vi "Initialize.vi"(8 "error in":errorcluster, 10 "parameters":variant, 11 "node in":refnum<class "CentralErrorHandler editor node.lvclass">) -> (0 "error out":errorcluster, 2 "summary":T2[](array[typedef]), 3 "data value reference":T1)   [LabVIEW 2017, in "CentralErrorHandler editor node.lvclass"]
doc: "Initializes the data of a node to its default state.\nThe object is not created inside of this VI, because it is created from a File depending on user selection."
uses:
  CentralErrorHandler editor node.lvclass
  C:/Program Files (x86)/National Instruments/LabVIEW 2017/vi.lib/NI/Configuration Framework/Node/NISE_CEF_Node.lvclass
  <vilib>/NI/Configuration Framework/Node/Summary.ctl
  <vilib>/NI/Configuration Framework/Node/NodeRef.ctl
  <vilib>/NI/Configuration Framework/Node/NISE_CEF_Node.lvclass
  module/configuration/CentralErrorHandler configuration.lvclass
  C:/Program Files (x86)/National Instruments/LabVIEW 2017/vi.lib/NI/Configuration Framework/serializable configuration/NISE_CEF_serializable configuration.lvclass
  <vilib>/NI/DCAF/Tag Editor Core/control module/editor node/control module editor.lvclass
  <vilib>/NI/Configuration Framework/serializable configuration/NISE_CEF_serializable configuration.lvclass
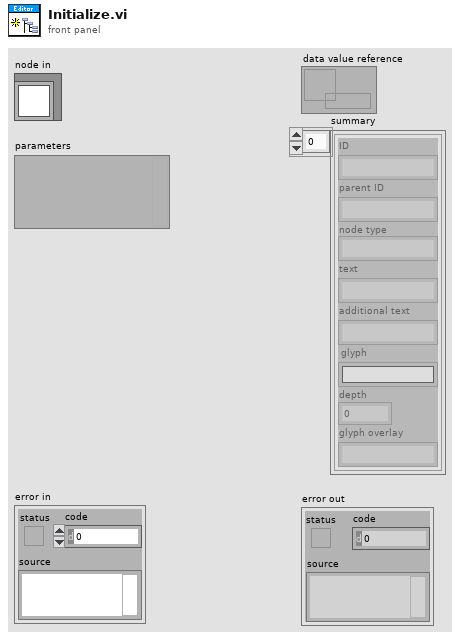
[diagram p1: front panel]
types:
  T1 = typedef "NISE_CEF_Node.lvclass/NodeRef.ctl" = refnum<data-value>
  T2 = typedef "NISE_CEF_Node.lvclass/Summary.ctl" = cluster{"ID":string, "parent ID":string, "node type":string, "text":string, "additional text":string, "glyph":string, "depth":i32, "glyph overlay":string}
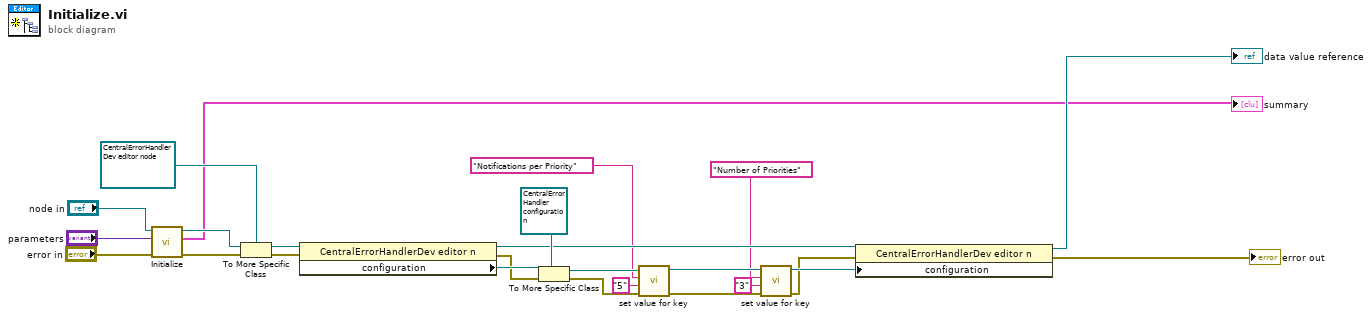
[diagram p0: block diagram]
diagram:
  n1 = call-parent "Initialize.vi"("error in"="error in", "parameters"="parameters", "node in"="node in") -> ("error out"=w8:errorcluster, "summary"=→"summary":T2[], "data value reference"=w6:T1)  [unwired: 6 in]
  n2 = To More Specific Class(target class=refnum<data-value> refnum ("data value reference"), reference=w6, error in=w8) -> (specific class reference=w4:refnum<data-value>, error out=w7:errorcluster)
  n3 = property class="CentralErrorHandlerDev editor n"(reference=w4, error in=w7) -> (reference out=w17:refnum<data-value>, error out=w23:errorcluster, "configuration"=w25:refnum<class "NISE_CEF_serializable configuration.lvclass">)
  n4 = To More Specific Class(target class=refnum<class "CentralErrorHandler configuration.lvclass"> refnum ("CentralErrorHandlerDev configuration"), reference=w25, error in=w23) -> (specific class reference=w22:refnum<class "CentralErrorHandler configuration.lvclass">, error out=w21:errorcluster)
  n5 = call-dynamic "set value for key.vi"("error in"=w21, "value"="5", "key"="Notifications per Priority", "fixed channel configuration in"=w22) -> ("error out"=w19:errorcluster, "fixed channel configuration out"=w20:refnum<class "CentralErrorHandler configuration.lvclass">)  [unwired: 6 in]
  n6 = call-dynamic "set value for key.vi"("error in"=w19, "value"="3", "key"="Number of Priorities" ("String"), "fixed channel configuration in"=w20) -> ("error out"=w16:errorcluster, "fixed channel configuration out"=w18:refnum<class "CentralErrorHandler configuration.lvclass">)  [unwired: 6 in]
  n7 = property class="CentralErrorHandlerDev editor n"(reference=w17, error in=w16, "configuration"=w18) -> (reference out=→"data value reference":refnum<data-value>, error out=→"error out":errorcluster)
